vi "Warning test.vi"(9 "Warning Instance":i32, 10 "Warnings Occured":i32[](array[numeric])) -> (2 "Warning Occured out":i32[](array[numeric]))   [LabVIEW 2013]
panel:
  in  "stop":bool
  out "Index Values":u32[](array[numeric])
  in  "Array 2":string[](array[string])
  out "Array":string[](array[string])
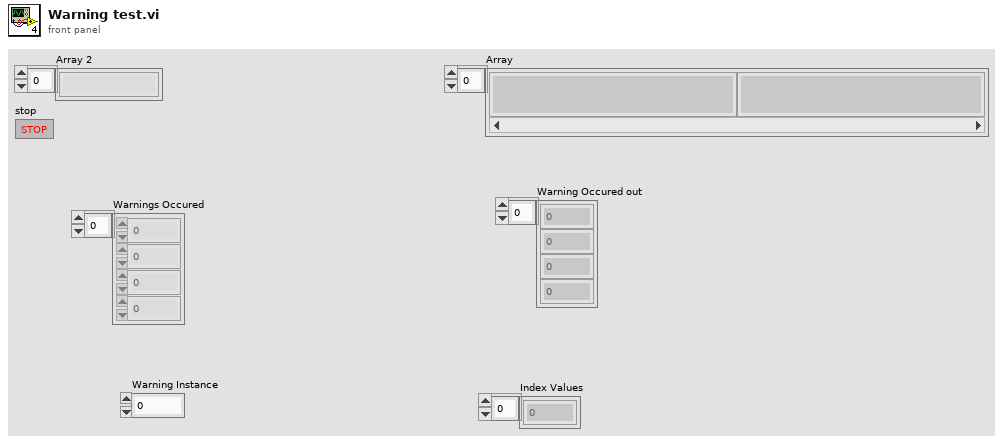
[diagram p1: front panel]
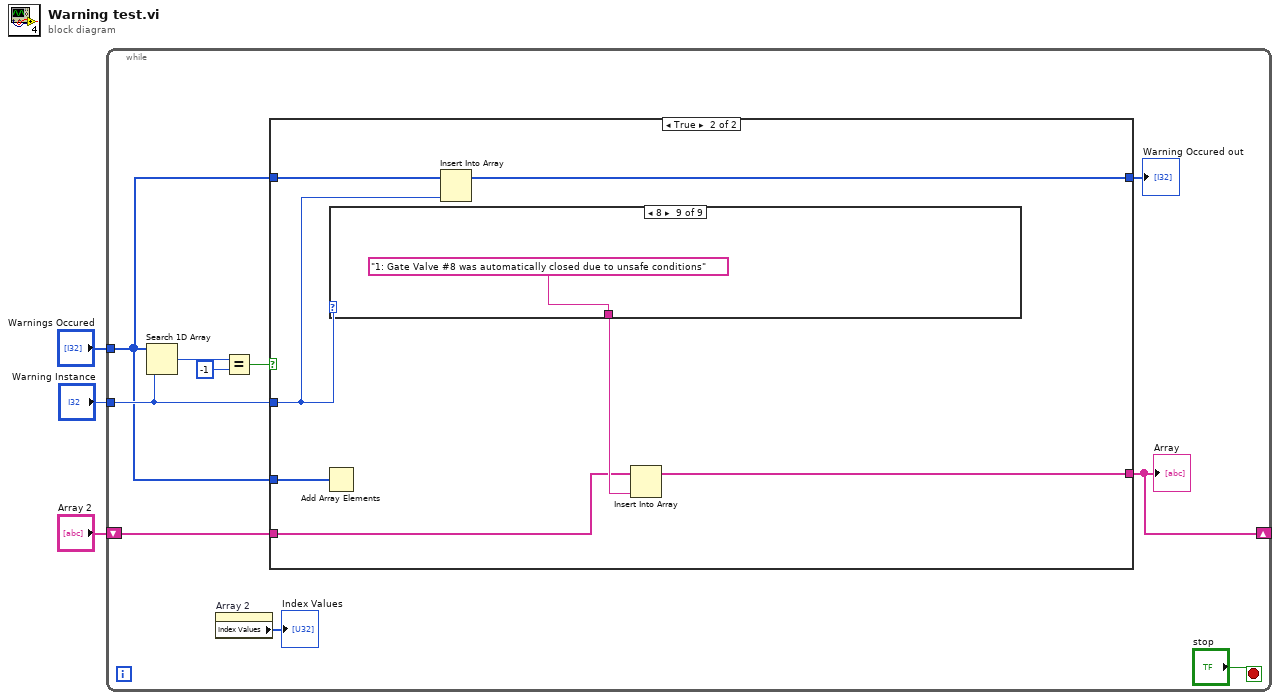
[diagram p0: block diagram]
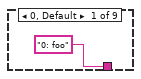
[diagram p3: hidden frame]
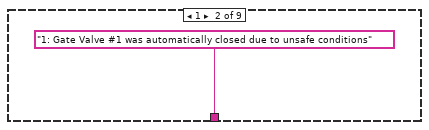
[diagram p4: hidden frame]
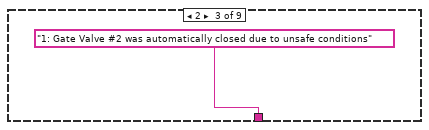
[diagram p5: hidden frame]
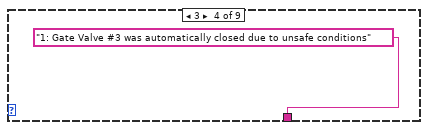
[diagram p6: hidden frame]
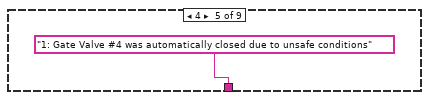
[diagram p7: hidden frame]
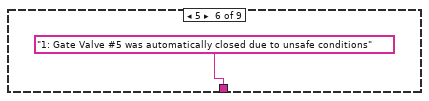
[diagram p8: hidden frame]
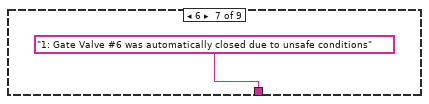
[diagram p9: hidden frame]
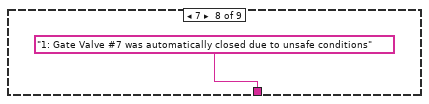
[diagram p10: hidden frame]
diagram:
  n1 = while {
    tunnel: "Warning Instance" -> [w10]
    tunnel: "Warnings Occured" -> [w8]
    shift-right: [w5] -> _
    shift-left: "Array 2" -> [w7]
    stop <- "stop" stop-if-true
    n2 = Search 1D Array(1D array=w8, element=w10) -> (index of element=w12:i32)  [unwired: 1 in]
    n3 = property on="Array 2" class="Arr (strict)"() -> ("Index Values"=→"Index Values":u32[])  [unwired: 2 in, 2 out]
    n4 = Equal?(x=w12, y=-1) -> (x = y?=w11:bool)
    n5 = case shown="True" w11 {
      tunnel: w10 -> [_ w22]
      tunnel: w8 -> [w15 w21]
      tunnel: [w15 w20] -> w9
      tunnel: w8 -> [_ w19]
      tunnel: [w14 w17] -> w5
      tunnel: w7 -> [w14 w16]
      frame False {
      }
      frame True {
        n6 = Add Array Elements(numeric array=w19) -> ()  [unwired: 1 out]
        n7 = case shown="8" w22 {
          tunnel: ["0: foo" "1: Gate Valve #1 was automatically closed due to unsafe conditions" "1: Gate Valve #2 was automatically closed due to unsafe conditions" "1: Gate Valve #3 was automatically closed due to unsafe conditions" "1: Gate Valve #4 was automatically closed due to unsafe conditions" "1: Gate Valve #5 was automatically closed due to unsafe conditions" "1: Gate Valve #6 was automatically closed due to unsafe conditions" "1: Gate Valve #7 was automatically closed due to unsafe conditions" "1: Gate Valve #8 was automatically closed due to unsafe conditions"] -> w18
          frame 0, Default {
          }
          frame 1 {
          }
          frame 2 {
          }
          frame 3 {
          }
          frame 4 {
          }
          frame 5 {
          }
          frame 6 {
          }
          frame 7 {
          }
          frame 8 {
          }
        }
        n8 = Insert Into Array(array=w21, new element=w22) -> (w20:i32[])  [unwired: 1 in]
        n9 = Insert Into Array(array=w16, new element=w18) -> (w17:string[])  [unwired: 1 in]
      }
    }
    "Warning Occured out" <- w9
    "Array" <- w5
  }
